vi "Arm Hardware.vi"(8 "error in (no error)":errorcluster, 9 "Request type":T1=enum."User command", 11 "DAQmx Digitizer in":refnum<class "DAQmx Synthesizer.lvclass">) -> (0 "error out":errorcluster, 3 "DAQmx Digitizer out":refnum<class "DAQmx Synthesizer.lvclass">)   [LabVIEW 2024, in "DAQmx Synthesizer.lvclass"]
uses:
  DAQmx Synthesizer.lvclass
  LabActor/Controllers/Process Controller/Request type.ctl
  DAQmx Digitizer/DAQmx Digitizer.lvclass
  DAQmx Synthesizer.lvclass/DAQmx Synthesizer.ctl
  <resource>/objmgr/daqmx.rc
  File/File Class/File.lvclass
  <vilib>/DAQmx/configure/trigger.llb/DAQmx Start Trigger (Digital Edge).vi
  <vilib>/DAQmx/write.llb/DAQmx Write (Analog 1D Wfm NChan NSamp).vi
  <vilib>/DAQmx/create/channels.llb/DAQmx Create Channel (AO-Voltage-Basic).vi
  <vilib>/DAQmx/configure/timing.llb/DAQmx Timing (Sample Clock).vi
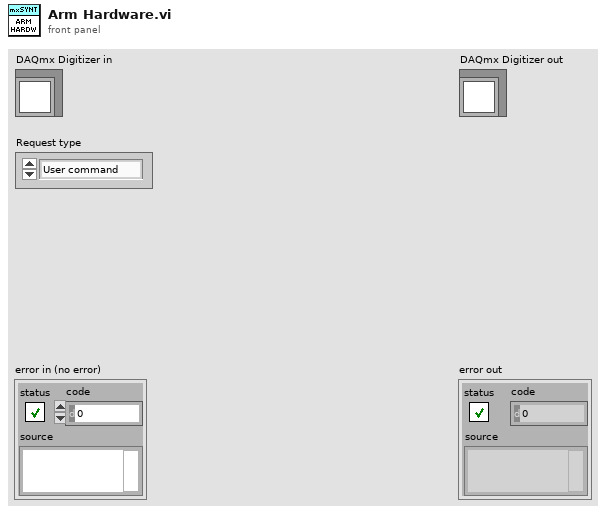
[diagram p1: front panel]
types:
  T1 = typedef "Request type.ctl" = enum16{"Process complete", "User command", "Auto-restart", "Error"}
  T2 = typedef "DAQmx Synthesizer Configuration.ctl" = cluster{"Channel names":string[], "Waveform file":path, "Ranges":dbl[], "Post-trigger delay":dbl, "Post-trigger duration":dbl, "Rate":dbl, "Re-name channels":string[], "Active channels":string, "External\nclock":bool, "Group name":string}
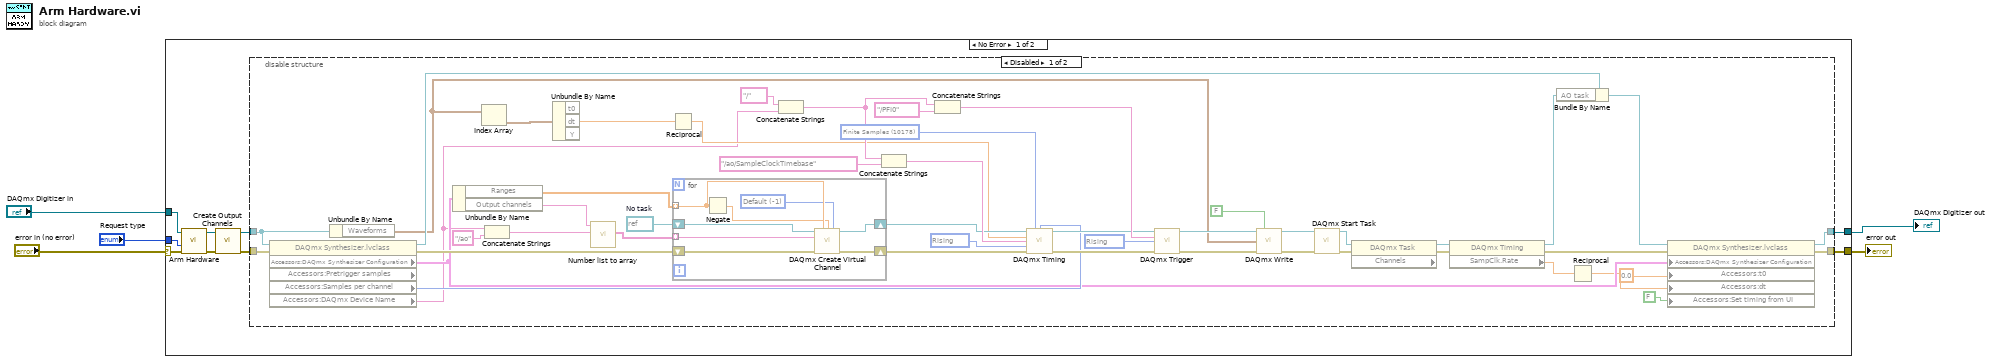
[diagram p0: block diagram]
diagram:
  n1 = case shown="No Error" "error in (no error)" {
    selector: "error in (no error)" -> [w12 w74]
    tunnel: [w13 w74] -> w4
    tunnel: [w14 w73] -> w2
    tunnel: "DAQmx Digitizer in" -> [w11 w73]
    tunnel: "Request type" -> [w10 _]
    frame No Error {
      n2 = call-parent "Arm Hardware.vi"("error in (no error)"=w12, "Request type"=w10, "DAQmx Digitizer in"=w11) -> ("error out"=w6:errorcluster, "DAQmx Digitizer out"=w9:refnum<class "DAQmx Synthesizer.lvclass">)  [unwired: 7 in]
      n3 = call-dynamic "Create Output Channels.vi"("error in (no error)"=w6, "DAQmx Lockin Digitizer Driver in"=w9) -> ("error out"=w7:errorcluster, "DAQmx Lockin Digitizer Driver out"=w8:refnum<class "DAQmx Synthesizer.lvclass">)  [unwired: 8 in]
      n4 = disable-structure shown="Disabled" {
        disable-tunnel: [w45 w72] -> w14
        disable-tunnel: [w44 w71] -> w13
        disable-tunnel: w7 -> [w16 w71]
        disable-tunnel: w8 -> [w15 w72]
        frame Disabled {
          w47 = refnum<k21> refnum  # No task
          w54 = 10280 items=["Rising"=10280, "Falling"=10171] ("active edge")
          w55 = 10178 items=["Finite Samples"=10178, "Continuous Samples"=10123, "Hardware Timed Single Point"=12522] ("sample mode")
          w62 = 10280 items=["Rising"=10280, "Falling"=10171] ("edge")
          n5 = property class="DAQmx Synthesizer.lvclass" props=["Accessors:DAQmx Synthesizer Configuration", "Accessors:Pretrigger samples", "Accessors:Samples per channel", "Accessors:DAQmx Device Name"](reference=w15, error in=w16) -> (reference out=w42:refnum<class "DAQmx Synthesizer.lvclass">, error out=w43:errorcluster, "Accessors:DAQmx Synthesizer Configuration"=w38:T2, "Accessors:Samples per channel"=w39:i32, "Accessors:DAQmx Device Name"=w17:tag)  [unwired: 1 out]
          n6 = Unbundle By Name(w15) -> ("Waveforms"=w21:waveform(dbl)[])
          n7 = Unbundle By Name(w38) -> ("Ranges"=w37:dbl[], "Output channels"=w50:string)
          n8 = Index Array(array=w21) -> (element=w28:waveform(dbl))  [unwired: 1 in]
          n9 = Concatenate Strings(w17, "/ao" ("string")) -> (w48:string)
          n10 = Unbundle By Name(w28) -> ("dt"=w27:dbl)  [unwired: 2 out]
          n11 = call "Number list to array.vi"("Full names prefix"=w48, "Number list"=w50) -> ("Full names"=w46:string[])  [unwired: 6 in, 3 out]
          n12 = Reciprocal(x=w27) -> (1/x=w26:dbl)
          n13 = for {
            tunnel: w46 -> [w70] mode=indexing
            tunnel: w37 -> [w68] mode=indexing
            shift-right: [w65] -> w61
            shift-left: w43 -> [w69]
            shift-right: [w66] -> w36
            shift-left: w47 -> [w63]
            w64 = -1 items=["Default"=-1, "RSE"=10083, "NRSE"=10078, "Differential"=10106, "Pseudodifferential"=12529] ("input terminal configuration")
            n14 = Negate(x=w68) -> (-x=w67:dbl)
            n15 = call-poly <vilib>:"DAQmx Create Virtual Channel.vi"("task in"=w63, "maximum value"=w68, "minimum value"=w67, "output terminal configuration"=w64, "physical channels"=w70, "error in"=w69) -> ("task out"=w66:refnum<k21>, "error out"=w65:errorcluster)  [unwired: 8 in]
          }
          n16 = Concatenate Strings(tag "/" ("string"), w17) -> (w29:string)
          n17 = Concatenate Strings(w29, tag "/ao/SampleClockTimebase" ("string")) -> (w53:string)
          n18 = Concatenate Strings(w29, tag "/PFI0" ("string")) -> (w59:string)
          n19 = call-poly <vilib>:"DAQmx Timing.vi"("task/channels in"=w36, "sample mode"=w55, "samples per channel"=w39, "rate"=w26, "source"=w53, "active edge"=w54, "error in"=w61) -> ("task out"=w57:refnum<k21>, "error out"=w58:errorcluster)  [unwired: 7 out]
          n20 = call-poly <vilib>:"DAQmx Trigger.vi"("task/channels in"=w57, "source"=w59, "edge"=w62, "error in"=w58) -> ("task out"=w25:refnum<k21>, "error out"=w23:errorcluster)  [unwired: 10 out]
          n21 = call-poly <vilib>:"DAQmx Write.vi"("task/channels in"=w25, "auto start"=FALSE, "data"=w21, "error in"=w23) -> ("task out"=w24:refnum<k21>, "error out"=w22:errorcluster)  [unwired: 9 in, 1 out]
          n22 = call <vilib>:"DAQmx Start Task.vi"("task/channels in"=w24, "error in"=w22) -> ("task out"=w52:refnum<k21>, "error out"=w51:errorcluster)  [unwired: 12 out]
          n23 = property class="DAQmx Task" props=["Channels"](reference=w52, error in=w51) -> (reference out=w41:refnum<k21>, error out=w40:errorcluster)  [unwired: 1 out]
          n24 = property class="DAQmx Timing"(reference=w41, error in=w40) -> (reference out=w18:refnum<k21>, error out=w34:errorcluster, "SampClk.Rate"=w35:dbl)
          n25 = Bundle By Name(cluster=w42, "AO task"=w18) -> (w60:refnum<class "DAQmx Synthesizer.lvclass">)
          n26 = Reciprocal(x=w35) -> (1/x=w33:dbl)
          n27 = property class="DAQmx Synthesizer.lvclass"(reference=w60, error in=w34, "Accessors:DAQmx Synthesizer Configuration"=w38, "Accessors:t0"=0.0, "Accessors:dt"=w33, "Accessors:Set timing from UI"=FALSE ("Set timing from UI")) -> (reference out=w45:refnum<class "DAQmx Synthesizer.lvclass">, error out=w44:errorcluster)
        }
        frame Enabled {
        }
      }
    }
    frame Error {
    }
  }
  "error out" <- w4
  "DAQmx Digitizer out" <- w2
